vi "Update Data Buffer.vi"(6 "gain":dbl, 8 "error in (no error)":errorcluster, 9 "dt":dbl, 10 "Data Buffer":T1, 11 "Application Manager in":refnum<class "Application Manager.lvclass">) -> (0 "error out":errorcluster, 3 "Application Manager out":refnum<class "Application Manager.lvclass">)   [LabVIEW 2020, in "Application Manager.lvlib" / "Application Manager.lvclass"]
uses:
  Application Manager.lvclass
  GPU FFT Calculator/GPU FFT Calculator/Data Source Buffer.ctl
  Application Manager.lvclass/Application Manager.ctl
  Calculation Worker/Calculation Worker Messages/Update Data Buffer Msg/Update Data Buffer Msg.lvclass/Update Data Buffer Msg.ctl
  <vilib>/ActorFramework/Message Enqueuer/Message Enqueuer.lvclass/Message Enqueuer.ctl
  Data Source/Data Source Messages/Continue Acquisition Msg/Continue Acquisition Msg.lvclass/Continue Acquisition Msg.ctl
  <vilib>/ActorFramework/Message Enqueuer/Enqueue.vi
  Calculation Worker/Calculation Worker Messages/Update Data Buffer Msg/Update Data Buffer Msg.lvclass
  C:/Program Files/National Instruments/LabVIEW 2026/vi.lib/ActorFramework/Message/Message.lvclass
  Data Source/Data Source Messages/Continue Acquisition Msg/Continue Acquisition Msg.lvclass
  <vilib>/ActorFramework/Message Priority Queue/Priority Enqueue.vi
  Data Source/Data Source/Data Source.lvclass
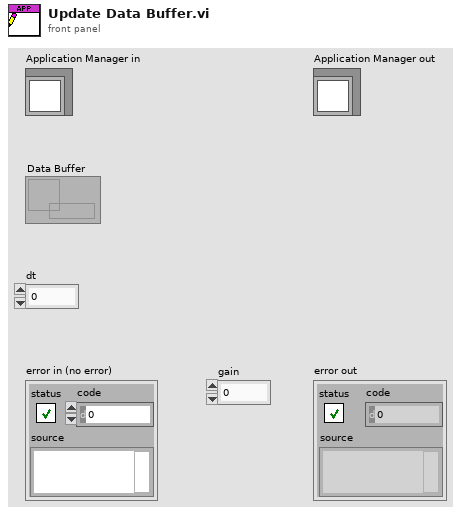
[diagram p1: front panel]
types:
  T1 = typedef "Data Source.lvlib/Data Source.lvclass/Data Source Buffer.ctl" = refnum<data-value>
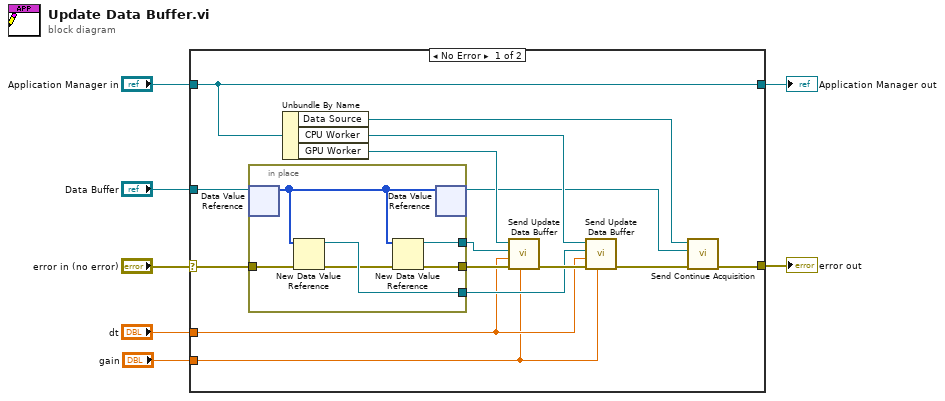
[diagram p0: block diagram]
diagram:
  n1 = case shown="No Error" "error in (no error)" {
    selector: "error in (no error)" -> [w17 w29]
    tunnel: [w10 w29] -> w6
    tunnel: [w22 w30] -> w4
    tunnel: "Application Manager in" -> [w22 w30]
    tunnel: "Data Buffer" -> [w16 _]
    tunnel: "dt" -> [w9 _]
    tunnel: "gain" -> [w8 _]
    frame No Error {
      n2 = in-place {
        in-place-border: [w28] -> w15
        in-place-border: [w27] -> w14
        in-place-border: [w25] -> w18
        in-place-border: w17 -> [w24]
        n3 = in-place-dvr #1(w16) -> (w23:i16[])  [unwired: 1 out]
        n4 = New Data Value Reference(data value=w23, error in=w24) -> (data value reference=w27:refnum<data-value>, error out=w26:errorcluster)
        n5 = New Data Value Reference(data value=w23, error in=w26) -> (data value reference=w28:refnum<data-value>, error out=w25:errorcluster)
        n6 = in-place-dvr #1(w23) -> (w11:T1)  [unwired: 1 out]
      }
      n7 = Unbundle By Name(w22) -> ("Data Source"=w12:refnum<class "Message Enqueuer.lvclass">, "CPU Worker"=w20:refnum<class "Message Enqueuer.lvclass">, "GPU Worker"=w21:refnum<class "Message Enqueuer.lvclass">)
      n8 = call "Send Update Data Buffer.vi"("gain"=w8, "error in (no error)"=w18, "dt"=w9, "Data Buffer"=w15, "Message Enqueuer"=w21) -> ("error out"=w19:errorcluster)  [unwired: 5 in, 1 out]
      n9 = call "Send Update Data Buffer.vi"("gain"=w8, "error in (no error)"=w19, "dt"=w9, "Data Buffer"=w14, "Message Enqueuer"=w20) -> ("error out"=w13:errorcluster)  [unwired: 5 in, 1 out]
      n10 = call "Send Continue Acquisition.vi"("error in (no error)"=w13, "Data Buffer"=w11, "Message Enqueuer"=w12) -> ("error out"=w10:errorcluster)  [unwired: 7 in, 1 out]
    }
    frame Error {
    }
  }
  "error out" <- w6
  "Application Manager out" <- w4
